vi "GLdrv_PUL_SCAL.vi"(0 "Connection ID":T1, 1 "Unit":string, 5 "CH":i32=1 min=1, 7 "Function":enum16{"ON", "OFF"}(ring), 9 "Scale In":string, 11 "error in (no error)":errorcluster, 12 "Scale Out":string, 13 "Query(f)":bool) -> (3 "Unit out":string, 4 "Connection ID Out":T1, 8 "Function out":enum16{"ON", "OFF"}(ring), 10 "Scale In out":string, 14 "Scale Out out":string, 15 "error out":errorcluster)   [LabVIEW 2017, in "GL860_Driver.lvlib"]
doc: "FUNC　スケーリングの機能の設定・参照\nOFF：　スケーリングをOffにします\nON：　スケールをOnにします\n例）　：PUL:CH1:SCAL:FUNC ON (パルスCH1のスケーリングを\nONにします)\nSET　スケーリングの入力側と出力側と単位の設定・参照\n例) PUL:CH1:SCAL:SET 1,100,”mL” (パルスCH1のスケーリン\nグを入力値を100倍にしたｍL単位に変換させます)\n例）　:PUL:CH2:SCAL:SET 10,5,\"Pa” (パルスCH2のスケーリン\nグを入力値を1/2倍にしたPa単位に変換させます)"
uses:
  GL860_Driver.lvlib
  ConnectionID.ctl
  GLdrv_RW.ctl
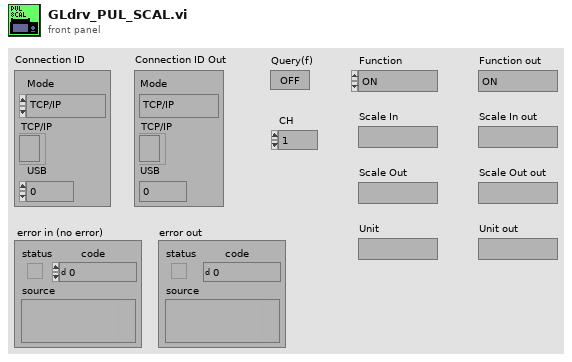
[diagram p1: front panel]
types:
  T1 = typedef "ConnectionID.ctl" = cluster{"Mode":enum16{"TCP/IP", "USB"}, "TCP/IP":refnum<k5>, "USB":i32}
  T2 = typedef "GLdrv_RW.ctl" = enum16{"Auto", "Read", "Write", "Buffer"}
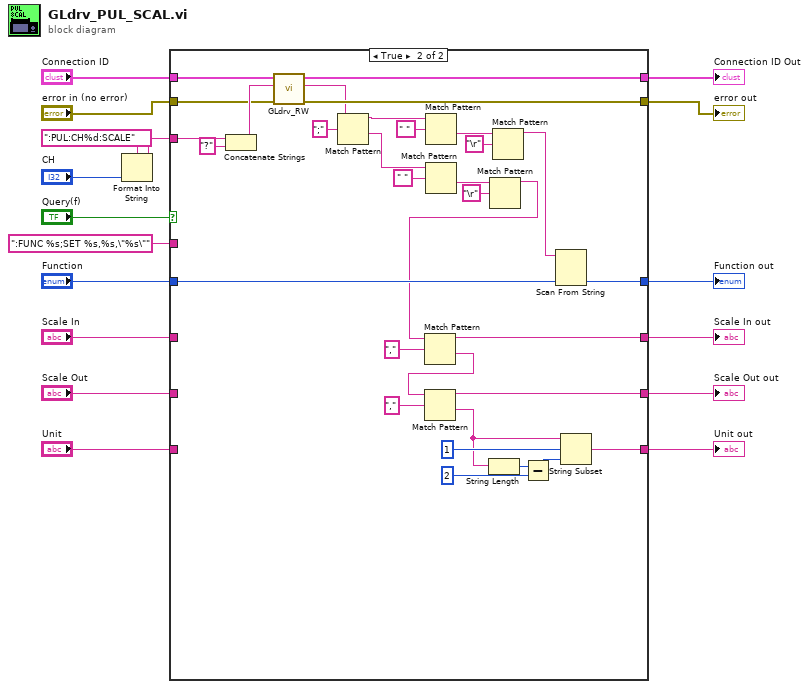
[diagram p0: block diagram]
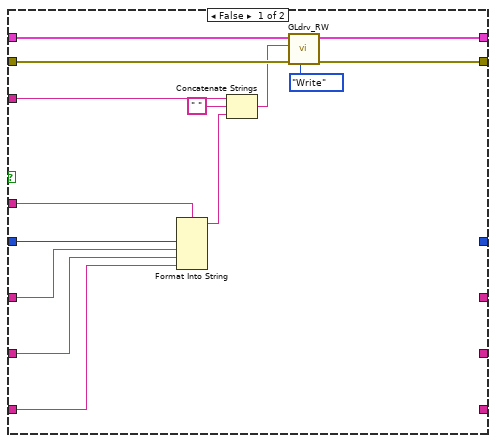
[diagram p2: hidden frame]
diagram:
  n1 = Format Into String(format string=":PUL:CH%d:SCALE" ("Command"), "CH") -> (resulting string=w11:string)  [unwired: 2 in, 1 out]
  n2 = case shown="TRUE" "Query(f)" {
    tunnel: w11 -> [w31 w63]
    tunnel: [w26 w57] -> w17
    tunnel: [w28 w60] -> w16
    tunnel: "Connection ID" -> [w29 w61]
    tunnel: "error in (no error)" -> [w27 w58]
    tunnel: "Function" -> [w22 w49]
    tunnel: ":FUNC %s;SET %s,%s,\"%s\"" ("Param") -> [w21 _]
    tunnel: "Scale In" -> [w20 _]
    tunnel: "Scale Out" -> [w19 _]
    tunnel: "Unit" -> [w18 _]
    tunnel: [_ w33] -> w5
    tunnel: [_ w32] -> w4
    tunnel: [_ w36] -> w3
    tunnel: [_ w35] -> w2
    frame False {
      n3 = Format Into String(format string=w21, w22, w20, w19, w18) -> (resulting string=w23:string)  [unwired: 2 in, 1 out]
      n4 = Concatenate Strings(w31, " " ("string"), w23) -> (w25:string)
      n5 = call "GLdrv_RW.vi"("Mode(read)"=GLdrv_RW."Write", "error in (no error)"=w27, "data in"=w25, "Connection ID"=w29) -> ("error out"=w26:errorcluster, "Connection ID Out"=w28:T1)  [unwired: 3 in, 3 out]
    }
    frame True {
      n6 = Concatenate Strings(w63, "?" ("string")) -> (w59:string)
      n7 = call "GLdrv_RW.vi"("error in (no error)"=w58, "data in"=w59, "Connection ID"=w61) -> ("error out"=w57:errorcluster, "data out"=w50:string, "Connection ID Out"=w60:T1)  [unwired: 4 in, 2 out]
      n8 = Match Pattern(string=w50, regular expression=";" ("search string/char (-)")) -> (before substring=w51:string, after substring=w34:string)  [unwired: 3 out]
      n9 = Match Pattern(string=w51, regular expression=" " ("search string/char (-)")) -> (after substring=w54:string)  [unwired: 4 out]
      n10 = Match Pattern(string=w34, regular expression=" " ("search string/char (-)")) -> (after substring=w46:string)  [unwired: 4 out]
      n11 = Match Pattern(string=w46, regular expression="\r") -> (before substring=w45:string)  [unwired: 4 out]
      n12 = Match Pattern(string=w45, regular expression=",") -> (before substring=w33:string, after substring=w44:string)  [unwired: 3 out]
      n13 = Match Pattern(string=w44, regular expression=",") -> (before substring=w32:string, after substring=w40:string)  [unwired: 3 out]
      n14 = String Length(string=w40) -> (length=w39:i32)
      n15 = Match Pattern(string=w54, regular expression="\r") -> (before substring=w53:string)  [unwired: 4 out]
      n16 = Subtract(x=w39, y=2) -> (x-y=w38:i32)
      n17 = Scan From String(input string=w53, default 1=w49) -> (output 1=w35:enum16{"ON", "OFF"})  [unwired: 3 in, 3 out]
      n18 = String Subset(string=w40, offset (0)=1, length (rest)=w38) -> (substring=w36:string)
    }
  }
  "Connection ID Out" <- w16
  "error out" <- w17
  "Function out" <- w2
  "Scale In out" <- w5
  "Scale Out out" <- w4
  "Unit out" <- w3
